vi "Delete Contents In Tree.vi"(8 "error in (no error)":errorcluster, 9 "Delete Activate Node(False)":bool, 10 "Node Name":string, 11 "Browers in":refnum<class "Browers Controller.lvclass">) -> (0 "error out":errorcluster, 3 "Browers out":refnum<class "Browers Controller.lvclass">)   [LabVIEW 2015, in "Browers Controller.lvclass"]
uses:
  Browers Controller.lvclass
  Browers Controller.lvclass/Browers Controller.ctl
  Brower View/Brower View.lvclass/Brower View.ctl
  MyTreeAPI/MyTreeAPI.lvclass
  Brower View/Brower View.lvclass
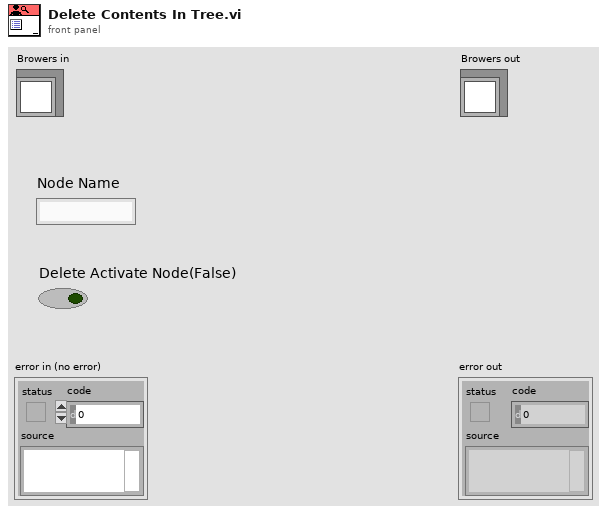
[diagram p1: front panel]
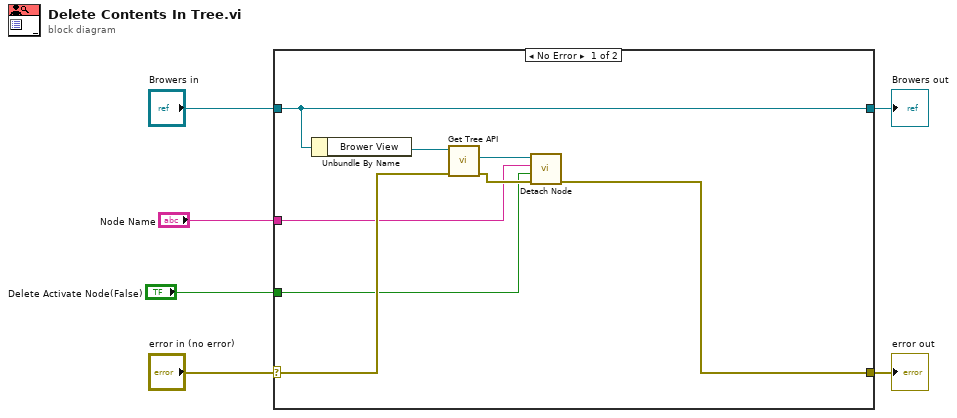
[diagram p0: block diagram]
diagram:
  n1 = case shown="No Error" "error in (no error)" {
    selector: "error in (no error)" -> [w12 w16]
    tunnel: [w9 w16] -> w5
    tunnel: [w14 w15] -> w3
    tunnel: "Browers in" -> [w14 w15]
    tunnel: "Node Name" -> [w8 _]
    tunnel: "Delete Activate Node(False)" -> [w7 _]
    frame No Error {
      n2 = Unbundle By Name(w14) -> ("Brower View"=w13:refnum<class "Brower View.lvclass">)
      n3 = call "Get Tree API.vi"("error in (no error)"=w12, "Brower View in"=w13) -> ("error out"=w10:errorcluster, "myTree.lvclass"=w11:refnum<class "MyTreeAPI.lvclass">)  [unwired: 7 in, 1 out]
      n4 = call "Detach Node.vi"("error in (no error)"=w10, "Delete Activate Node(False)"=w7, "Node Name"=w8, "TREE in"=w11) -> ("error out"=w9:errorcluster)  [unwired: 6 in, 1 out]
    }
    frame Error {
    }
  }
  "error out" <- w5
  "Browers out" <- w3
